vi "MoveForwardAndStraight.vi"(4 "Loop Timer":i32=20, 6 "Time to stop":i32=300, 8 "Distance":dbl, 9 "Encoder Left":dbl, 10 "Encoder Right":dbl, 11 "Yaw":dbl) -> (0 "Finished distance":bool, 1 "Both finished":bool, 2 "Direction":dbl, 3 "Trottle":dbl)   [LabVIEW 2019]
panel:
  in  "RangeGyro":cluster{"output high":dbl, "output low":dbl}={"output high"=0.3, "output low"=-0.3} {"output low" format="%.2f"; "output high" format="%.2f"}
  in  "GainsGyro":T1={"proportional gain (Kc)"=1.0, "integral time (Ti, min)"=0.01, "derivative time (Td, min)"=0.0} {"derivative time (Td, min)" format="%.3f"; "integral time (Ti, min)" format="%.3f"; "proportional gain (Kc)" format="%.3f"}
  in  "Range":cluster{"output high":dbl, "output low":dbl}={"output high"=0.95, "output low"=-0.4} {"output low" format="%.2f"; "output high" format="%.2f"}
  in  "Gains":T1={"proportional gain (Kc)"=1.0, "integral time (Ti, min)"=0.01, "derivative time (Td, min)"=0.0} {"derivative time (Td, min)" format="%.3f"; "integral time (Ti, min)" format="%.3f"; "proportional gain (Kc)" format="%.3f"}
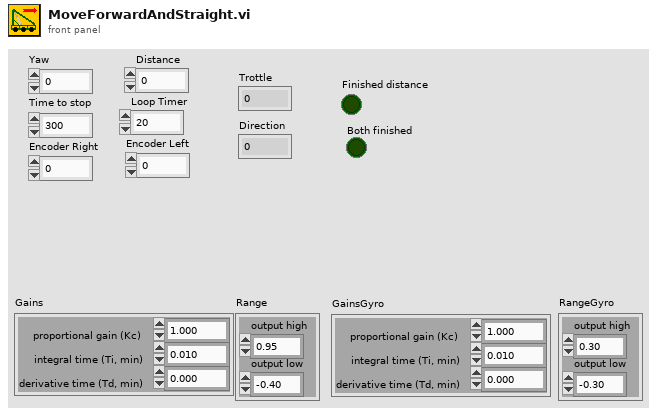
[diagram p1: front panel]
types:
  T1 = cluster{"proportional gain (Kc)":dbl, "integral time (Ti, min)":dbl, "derivative time (Td, min)":dbl}
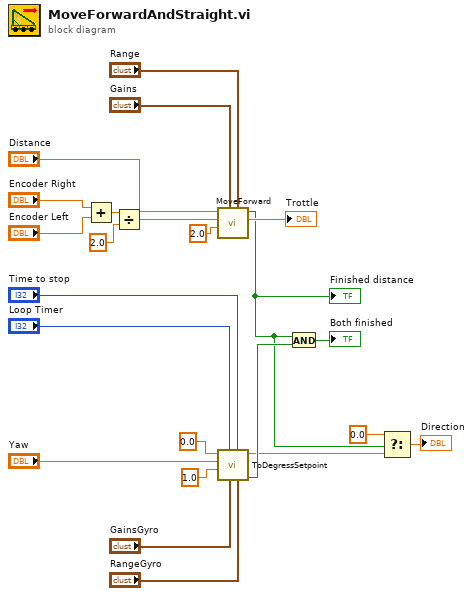
[diagram p0: block diagram]
diagram:
  n1 = Add(x="Encoder Right", y="Encoder Left") -> (x+y=w20:dbl)
  n2 = Divide(x=w20, y=2.0) -> (x/y=w18:dbl)
  n3 = call "MoveForward.vi"("Range"="Range", "Gains"="Gains", "Precision"=2.0, "Encoder Count"=w18, "Distance"="Distance") -> ("Output"=→"Trottle":dbl, "Finished?"=w5:bool)  [unwired: 5 in]
  "Finished distance" <- w5
  n4 = call "ToDegressSetpoint.vi"("Range"="RangeGyro", "Delay After"="Time to stop", "Gains"="GainsGyro", "Loop Wait Delay"="Loop Timer", "Precision"=1.0, "Yaw"="Yaw", "Setpoint (degress)"=0.0) -> ("Finished?"=w15:bool, "Output"=w8:dbl)  [unwired: 3 in]
  n5 = And(x=w5, y=w15) -> (x .and. y?=→"Both finished":bool)
  n6 = Select(t=0.0, s=w5, f=w8) -> (s? t:f=→"Direction":dbl)
